vi "Read structureDiagrams.vi"(8 "error in (no error)":errorcluster, 11 "Structure In":refnum<class "Structure.lvclass">) -> (0 "error out":errorcluster, 2 "strctureDiagrams":refnum<class "AbstractDiagram.lvclass">[](array[class]), 3 "Structure Out":refnum<class "Structure.lvclass">)   [LabVIEW 2023, in "TLC_Scripto.lvlib" / "Structure.lvclass"]
uses:
  GObject/Read GObjectRef.vi
  Structure.lvclass
  Structure.lvclass/Structure.ctl
  AbstractDiagram/AbstractDiagram.lvclass
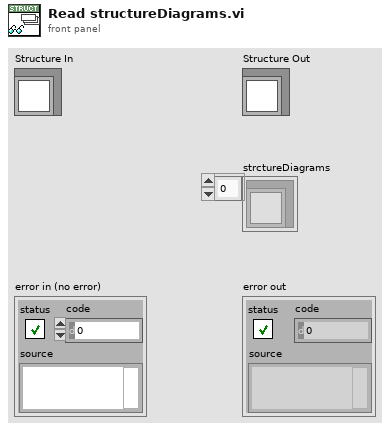
[diagram p1: front panel]
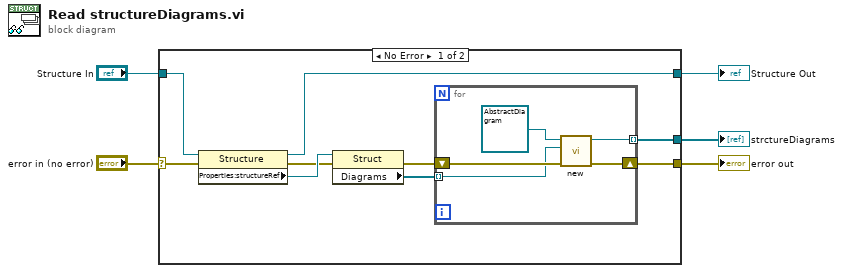
[diagram p0: block diagram]
diagram:
  n1 = case shown="No Error" "error in (no error)" {
    selector: "error in (no error)" -> [w12 w21]
    tunnel: [w14 w21] -> w1
    tunnel: [w11 w20] -> w3
    tunnel: "Structure In" -> [w10 w20]
    tunnel: [w13 _] -> w2
    frame No Error {
      n2 = property class="Structure"(reference=w10, error in=w12) -> (reference out=w11:refnum<class "Structure.lvclass">, error out=w8:errorcluster, "Properties:structureRef"=w9:refnum<vi>)
      n3 = property class="Struct"(reference=w9, error in=w8) -> (error out=w7:errorcluster, "Diagrams"=w6:refnum<vi>[])  [unwired: 1 out]
      n4 = for {
        shift-right: [w18] -> w14
        shift-left: w7 -> [w19]
        tunnel: [w17] -> w13 mode=indexing
        tunnel: w6 -> [w15] mode=indexing
        n5 = call-dynamic "new.vi"("Error In"=w19, "ref"=w15, "Generic In"=refnum<class "AbstractDiagram.lvclass"> refnum ("TLC_Scripto.lvlib:AbstractDiagram.lvclass")) -> ("Error Out"=w18:errorcluster, "Generic Out"=w17:refnum<class "AbstractDiagram.lvclass">)  [unwired: 7 in]
      }
    }
    frame Error {
    }
  }
  "error out" <- w1
  "Structure Out" <- w3
  "strctureDiagrams" <- w2
